vi "Vision Processing.vi"(4 "error in (no error)":errorcluster, 7 "Image Size":T1=enum."320x240") -> ()   [LabVIEW 2016]
doc: "This VI runs in parallel to other tasks. It gets images from the camera, processes them for color or shape and use that information to affect robot behavior."
uses:
  <vilib>/Rock Robotics/WPI/Camera/WPI_CameraImageSize.ctl
  <vilib>/Rock Robotics/WPI/Camera/WPI_CameraFrameRate.ctl
  <vilib>/Rock Robotics/WPI/Camera/WPI_CameraWhite Balance Values.ctl
  <vilib>/Rock Robotics/WPI/Camera/WPI_CameraExposure Values.ctl
  Robot Global Data.vi
panel:
  in  "Image Size 2":T1
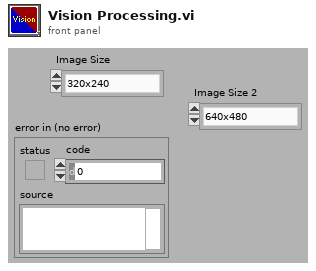
[diagram p1: front panel]
types:
  T1 = typedef "WPI_CameraImageSize.ctl" = enum16{"640x480", "320x240", "160x120", "Custom"}
  T2 = typedef "Image Type" = u32
  T3 = typedef "WPI_CameraFrameRate.ctl" = u32
  T4 = typedef "WPI_CameraExposure Values.ctl" = enum16{"Auto", "Flicker-free 50 Hz", "Flicker-free 60 Hz", "Hold current", "Custom"}
  T5 = typedef "WPI_CameraWhite Balance Values.ctl" = enum16{"Auto", "Fixed indoor", "Fixed outdoor 1", "Fixed outdoor 2", "Fixed fluorescent 1", "Fixed fluorescent 2", "Hold current", "Custom"}
  T6 = typedef "WPI_CameraDevRef.ctl" = cluster{"Camera Address":string, "CameraStatus":errorcluster}
  T7 = typedef "IMAQ Image.ctl" = refnum<image>
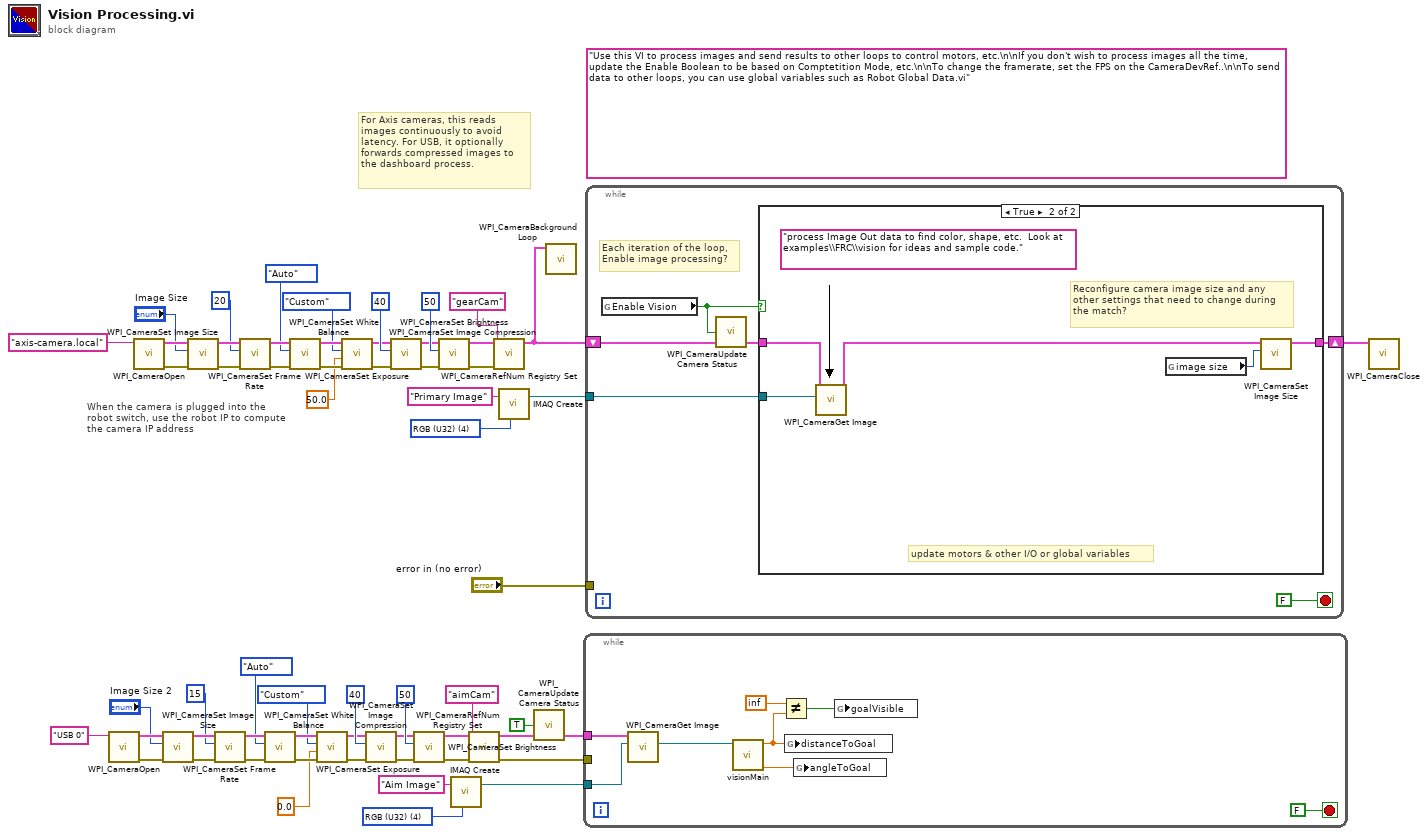
[diagram p0: block diagram]
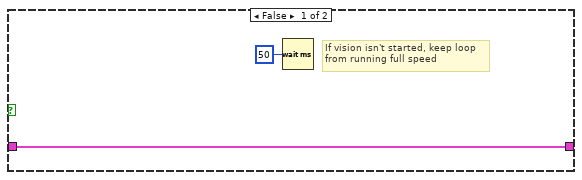
[diagram p2: hidden frame]
diagram:
  w7 = T2 4 items=["Grayscale (U8)", "Grayscale (I16)", "Grayscale (SGL)", "Complex (CSG)", "RGB (U32)", "HSL (U32)", "RGB (U64)"] ("Image Type")
  (unwired) "Use this VI to process images and send results to other loops to control motors, etc.\n\nIf you don't wish to process images all the time, update the Enable Boolean to be based on Comptetition Mode, etc.\n\nTo change the framerate, set the FPS on the CameraDevRef..\n\nTo send data to other loops, you can use global variables such as Robot Global Data.vi"
  w59 = T2 4 items=["Grayscale (U8)", "Grayscale (I16)", "Grayscale (SGL)", "Complex (CSG)", "RGB (U32)", "HSL (U32)", "RGB (U64)"] ("Image Type")
  # "When the camera is plugged into the\nrobot switch, use the robot IP to compute\nthe camera IP address"
  # "For Axis cameras, this reads\nimages continuously to avoid\nlatency. For USB, it optionally\nforwards compressed images to\nthe dashboard process."
  n1 = call <vilib>:"WPI_CameraOpen.vi"("Camera Address"="USB 0" ("format string")) -> ("error out"=w21:errorcluster, "CameraDevRef"=w22:T6)  [unwired: 1 in, 8 out]
  n2 = call <vilib>:"WPI_CameraOpen.vi"("Camera Address"="axis-camera.local" ("format string")) -> ("error out"=w47:errorcluster, "CameraDevRef"=w48:T6)  [unwired: 1 in, 8 out]
  n3 = call <vilib>:"WPI_CameraSet Image Size.vi"("error in (no error)"=w21, "Image Size"="Image Size 2", "CameraDevRef"=w22) -> ("error out"=w20:errorcluster, "CameraDevRef Out"=w23:T6)  [unwired: 1 in, 6 out]
  n4 = call <vilib>:"WPI_CameraSet Image Size.vi"("error in (no error)"=w47, "Image Size"="Image Size", "CameraDevRef"=w48) -> ("error out"=w46:errorcluster, "CameraDevRef Out"=w49:T6)  [unwired: 1 in, 6 out]
  n5 = call <vilib>:"WPI_CameraSet Frame Rate.vi"("error in (no error)"=w20, "Frame Rate (fps)"=T3 15, "CameraDevRef"=w23) -> ("error out"=w19:errorcluster, "CameraDevRef Out"=w25:T6)  [unwired: 7 out]
  n6 = call <vilib>:"WPI_CameraSet Frame Rate.vi"("error in (no error)"=w46, "Frame Rate (fps)"=T3 20, "CameraDevRef"=w49) -> ("error out"=w45:errorcluster, "CameraDevRef Out"=w51:T6)  [unwired: 7 out]
  n7 = call <vilib>:"WPI_CameraSet White Balance.vi"("error in (no error)"=w19, "White Balance"=WPI_CameraWhite_Balance_Values."Auto", "CameraDevRef"=w25) -> ("error out"=w18:errorcluster, "CameraDevRef Out"=w24:T6)  [unwired: 1 in, 6 out]
  n8 = call <vilib>:"WPI_CameraSet White Balance.vi"("error in (no error)"=w45, "White Balance"=WPI_CameraWhite_Balance_Values."Auto", "CameraDevRef"=w51) -> ("error out"=w44:errorcluster, "CameraDevRef Out"=w50:T6)  [unwired: 1 in, 6 out]
  n9 = call <vilib>:"WPI_CameraSet Exposure.vi"("error in (no error)"=w18, "Exposure (%)"=0.0, "Exposure"=WPI_CameraExposure_Values."Custom", "CameraDevRef"=w24) -> ("error out"=w17:errorcluster, "CameraDevRef Out"=w27:T6)  [unwired: 6 out]
  n10 = call <vilib>:"WPI_CameraSet Exposure.vi"("error in (no error)"=w44, "Exposure (%)"=50.0, "Exposure"=WPI_CameraExposure_Values."Custom", "CameraDevRef"=w50) -> ("error out"=w43:errorcluster, "CameraDevRef Out"=w53:T6)  [unwired: 6 out]
  n11 = call <vilib>:"WPI_CameraSet Image Compression.vi"("error in (no error)"=w17, "Compression"=40, "CameraDevRef"=w27) -> ("error out"=w16:errorcluster, "CameraDevRef Out"=w26:T6)  [unwired: 7 out]
  n12 = call <vilib>:"WPI_CameraSet Image Compression.vi"("error in (no error)"=w43, "Compression"=40, "CameraDevRef"=w53) -> ("error out"=w42:errorcluster, "CameraDevRef Out"=w52:T6)  [unwired: 7 out]
  n13 = call <vilib>:"WPI_CameraSet Brightness.vi"("error in (no error)"=w16, "Brightness"=50, "CameraDevRef"=w26) -> ("error out"=w14:errorcluster, "CameraDevRef Out"=w15:T6)  [unwired: 7 out]
  n14 = call <vilib>:"WPI_CameraSet Brightness.vi"("error in (no error)"=w42, "Brightness"=50, "CameraDevRef"=w52) -> ("error out"=w40:errorcluster, "CameraDevRef Out"=w41:T6)  [unwired: 7 out]
  n15 = call "IMAQ Create"("Image Name"="Aim Image", "Image Type"=w7) -> ("New Image"=w2:T7)  [unwired: 2 in, 2 out]
  n16 = call <vilib>:"WPI_CameraRefNum Registry Set.vi"("error in (no error)"=w14, "refnum name"="aimCam", "CameraDevRef"=w15) -> ("error out"=w1:errorcluster, "CameraDevRef"=w5:T6)  [unwired: 1 in, 6 out]
  n17 = call <vilib>:"WPI_CameraRefNum Registry Set.vi"("error in (no error)"=w40, "refnum name"="gearCam", "CameraDevRef"=w41) -> ("CameraDevRef"=w36:T6)  [unwired: 1 in, 7 out]
  n18 = call "IMAQ Create"("Image Name"="Primary Image", "Image Type"=w59) -> ("New Image"=w57:T7)  [unwired: 2 in, 2 out]
  n19 = call <vilib>:"WPI_CameraUpdate Camera Status.vi"("CameraDevRef In"=w5, "Enable Vision"=TRUE) -> ("CameraDevRef Out"=w3:T6)  [unwired: 3 in]
  n20 = call <vilib>:"WPI_CameraBackground Loop.vi"("CameraDevRef"=w36) -> ()  [unwired: 11 in]
  n21 = while {
    tunnel: w3 -> [w62]
    tunnel: w2 -> [w61]
    tunnel: w1 -> [_]
    stop <- FALSE stop-if-true
    n22 = call <vilib>:"WPI_CameraGet Image.vi"("Image"=w61, "CameraDevRef"=w62) -> ("Image Out"=w60:T7)  [unwired: 1 in, 8 out]
    n23 = call "visionMain.vi"("camImage"=w60) -> ("angle (deg)"=w64:dbl, "distance (ft)"=w66:dbl)  [unwired: 9 in]
    n24 = Not Equal?(x=inf, y=w66) -> (x != y?=w67:bool)
    n25 = global write "Robot Global Data.vi" "distanceToGoal"(w66) -> ()
    n26 = global write "Robot Global Data.vi" "angleToGoal"(w64) -> ()
    n27 = global write "Robot Global Data.vi" "goalVisible"(w67) -> ()
  }
  n28 = while {
    shift-right: [w72] -> w34
    shift-left: w36 -> [w70]
    tunnel: w57 -> [w71]
    tunnel: "error in (no error)" -> [_]
    stop <- FALSE stop-if-true
    # "Each iteration of the loop,\nEnable image processing?"
    n29 = global read "Robot Global Data.vi" "Enable Vision"() -> (w68:bool)
    n30 = call <vilib>:"WPI_CameraUpdate Camera Status.vi"("CameraDevRef In"=w70, "Enable Vision"=w68) -> ("CameraDevRef Out"=w69:T6)  [unwired: 3 in]
    n31 = case shown="True" w68 {
      tunnel: w71 -> [_ w79]
      tunnel: [w75 w80] -> w72
      tunnel: w69 -> [w75 w77]
      frame False {
        # "If vision isn't started, keep loop\nfrom running full speed"
        n32 = Wait (ms)(milliseconds to wait=u32 50) -> ()  [unwired: 1 out]
      }
      frame True {
        (unwired) "process Image Out data to find color, shape, etc.  Look at examples\\FRC\\vision for ideas and sample code."
        # "update motors & other I/O or global variables"
        # "Reconfigure camera image size and any\nother settings that need to change during\nthe match?"
        n33 = call <vilib>:"WPI_CameraGet Image.vi"("Image"=w79, "CameraDevRef"=w77) -> ("CameraDevRef Out"=w76:T6)  [unwired: 1 in, 8 out]
        n34 = global read "Robot Global Data.vi" "image size"() -> (w78:T1)
        n35 = call <vilib>:"WPI_CameraSet Image Size.vi"("Image Size"=w78, "CameraDevRef"=w76) -> ("CameraDevRef Out"=w80:T6)  [unwired: 2 in, 7 out]
      }
    }
  }
  n36 = call <vilib>:"WPI_CameraClose.vi"("CameraDevRef"=w34) -> ()  [unwired: 1 in, 10 out]
